vi "Offset.vi"(7 "Raw Data Waveform":T1, 10 "Offset":i32, 11 "(WavIndex_Pointer)":refnum<class "WavIndex_Pointer.lvclass">) -> (3 "(WavIndex_Pointer) Out":refnum<class "WavIndex_Pointer.lvclass">)   [LabVIEW 2024, in "WavIndex_Pointer.lvclass"]
uses:
  WavIndex_Pointer.lvclass
  Universal Controls/Waveform_Data.ctl
  WavIndex_Pointer.lvclass/WavIndex_Pointer.ctl
  Index_Pointer/Index_Pointer.lvclass
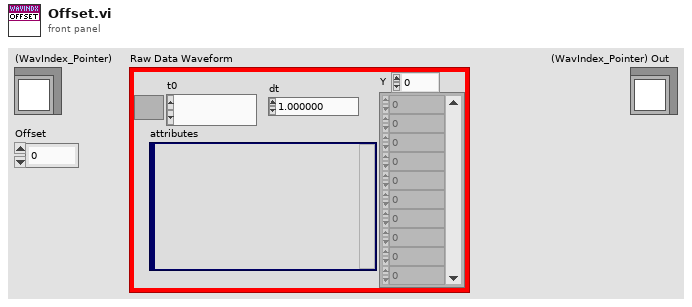
[diagram p1: front panel]
types:
  T1 = typedef "Waveform_Data.ctl" = waveform(dbl)
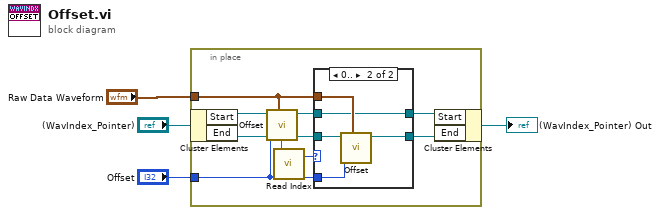
[diagram p0: block diagram]
diagram:
  n1 = in-place {
    in-place-border: "Offset" -> [w11]
    in-place-border: "Raw Data Waveform" -> [w7]
    n2 = in-place-cluster #1("(WavIndex_Pointer)") -> ("Start"=w10:refnum<class "Index_Pointer.lvclass">, "End"=w9:refnum<class "Index_Pointer.lvclass">)
    n3 = call-dynamic "Offset.vi"("Raw Data Waveform"=w7, "Offset"=w11, "(Index_Pointer)"=w10) -> ("(Index_Pointer) Out"=w6:refnum<class "Index_Pointer.lvclass">)  [unwired: 8 in]
    n4 = call "Read Index.vi"("Index_Pointer)"=w9) -> ("Index Out"=w8:i32)  [unwired: 2 in]
    n5 = case shown="0.." w8 {
      tunnel: [w14 w19] -> w12
      tunnel: w11 -> [_ w18]
      tunnel: w9 -> [w14 w17]
      tunnel: w7 -> [_ w16]
      tunnel: [w13 w15] -> w5
      tunnel: w6 -> [w13 w15]
      frame ..-1 {
      }
      frame 0.. {
        n6 = call-dynamic "Offset.vi"("Raw Data Waveform"=w16, "Offset"=w18, "(Index_Pointer)"=w17) -> ("(Index_Pointer) Out"=w19:refnum<class "Index_Pointer.lvclass">)  [unwired: 8 in]
      }
    }
    n7 = in-place-cluster #1("Start"=w5, "End"=w12) -> (→"(WavIndex_Pointer) Out":refnum<class "WavIndex_Pointer.lvclass">)
  }
